vi "Create Types.vi"(8 "error in (no error)":errorcluster, 11 "protoFile ref in":u64) -> (0 "error out":errorcluster, 2 "Enum Parameters":T4[](array[typedef]), 3 "Message Parameters":T5[](array[typedef]))   [LabVIEW 2019, in "gRPC Template Creation Utility.lvlib"]
uses:
  gRPC Template Creation Utility.lvlib
  TypeDefs/Message Metadata (Scripting).ctl
  TypeDefs/Message Element Metadata (Scripting).ctl
  TypeDefs/Message Element Type.ctl
  TypeDefs/Enum Metadata (Scripting).ctl
  TypeDefs/Oneof Metadata.ctl
panel:
  out "Oneof Parameters":T1[](array[typedef])
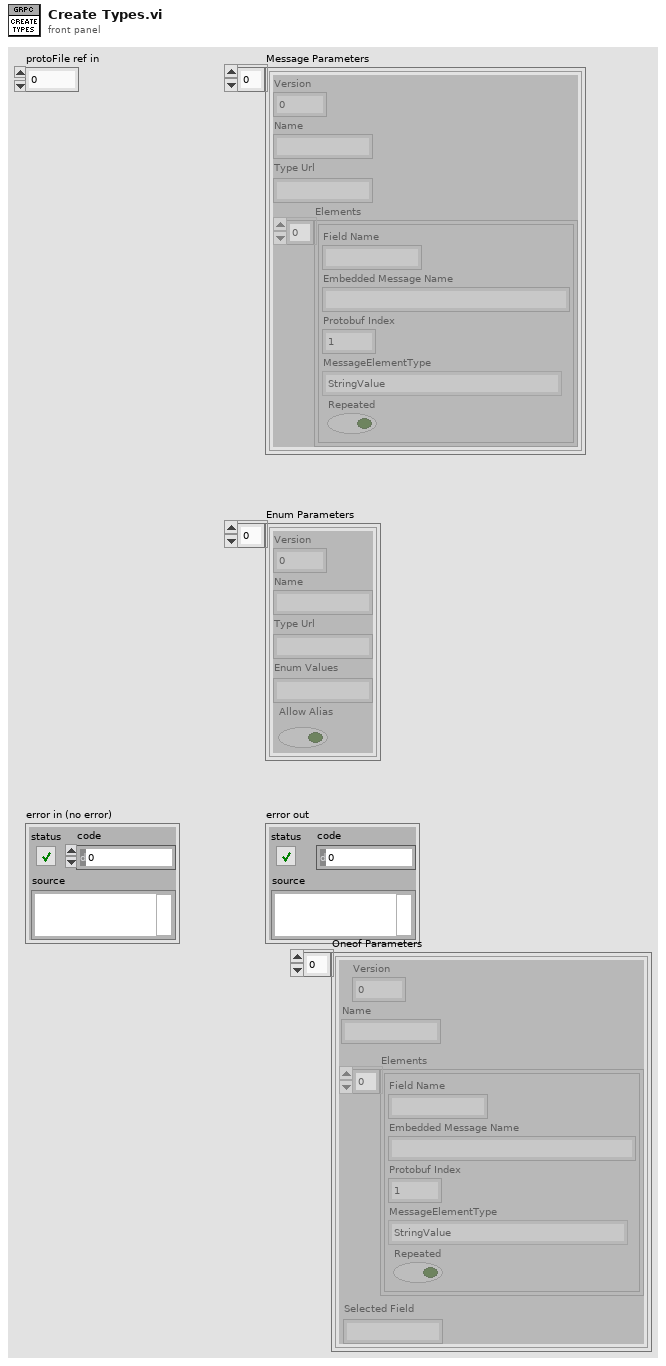
[diagram p1: front panel]
types:
  T1 = typedef "gRPC Template Creation Utility.lvlib/Oneof Metadata.ctl" = cluster{"Version":i32, "Name":string, "Elements":T2[], "Selected Field":string}
  T2 = typedef "gRPC Template Creation Utility.lvlib/Message Element Metadata (Scripting).ctl" = cluster{"Field Name":string, "Embedded Message Name":string, "Protobuf Index":i32, "MessageElementType":T3, "Repeated":bool}
  T3 = typedef "gRPC Template Creation Utility.lvlib/Message Element Type.ctl" = enum32{"Int32Value", "FloatValue", "DoubleValue", "BoolValue", "StringValue", "MessageValue", "Int64Value", "UInt32Value", "UInt64Value", "EnumValue", "Bytes", "Fixed64", "Fixed32", "SFixed64", "SFixed32", "SInt64", "SInt32", "Oneof"}
  T4 = typedef "gRPC Template Creation Utility.lvlib/Enum Metadata (Scripting).ctl" = cluster{"Version":i32, "Name":string, "Type Url":string, "Enum Values":string, "Allow Alias":bool}
  T5 = typedef "gRPC Template Creation Utility.lvlib/Message Metadata (Scripting).ctl" = cluster{"Version":i32, "Name":string, "Type Url":string, "Elements":T2[]}
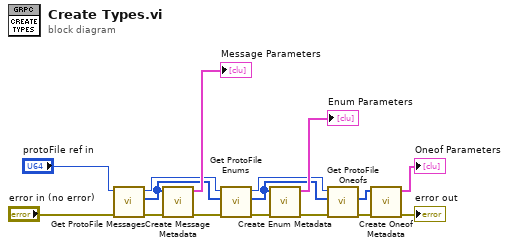
[diagram p0: block diagram]
diagram:
  n1 = call "Get ProtoFile Messages.vi"("error in (no error)"="error in (no error)", "Protofile ref in"="protoFile ref in") -> ("error out"=w11:errorcluster, "ProtoFile Messages"=w15:u64[], "Protofile ref out"=w14:u64)  [unwired: 7 in]
  n2 = call "Create Message Metadata.vi"("error in (no error)"=w11, "ProtoFile Messages"=w15) -> ("error out"=w9:errorcluster, "Message Parameters"=→"Message Parameters":T5[])  [unwired: 8 in]
  n3 = call "Get ProtoFile Enums.vi"("error in (no error)"=w9, "ProtoFile Messages"=w15, "Protofile ref in"=w14) -> ("error out"=w10:errorcluster, "ProtoFile Enums"=w6:u64[], "Protofile ref out"=w7:u64)  [unwired: 6 in]
  n4 = call "Create Enum Metadata.vi"("error in (no error)"=w10, "ProtoFile Enums"=w6) -> ("error out"=w5:errorcluster, "Enum Parameters"=→"Enum Parameters":T4[])  [unwired: 8 in]
  n5 = call "Get ProtoFile Oneofs.vi"("error in (no error)"=w5, "ProtoFile Messages"=w6, "Protofile ref in"=w7) -> ("error out"=w3:errorcluster, "ProtoFile Oneofs"=w4:u64[])  [unwired: 6 in, 1 out]
  n6 = call "Create Oneof Metadata.vi"("error in (no error)"=w3, "ProtoFile Oneofs"=w4) -> ("error out"=→"error out":errorcluster, "Oneof Parameters"=→"Oneof Parameters":T1[])  [unwired: 8 in]
